vi "Elevator Bang Bang (before rewrite).vi"(8 "Hold Up Mode":bool, 9 "Top":bool, 10 "Middle":bool, 11 "Bottom":bool) -> (3 "in range":bool)   [LabVIEW 2014]
uses:
  Robot Global Data.vi
panel:
  out "Pot Value":dbl
  in  "Last Fed Value":dbl
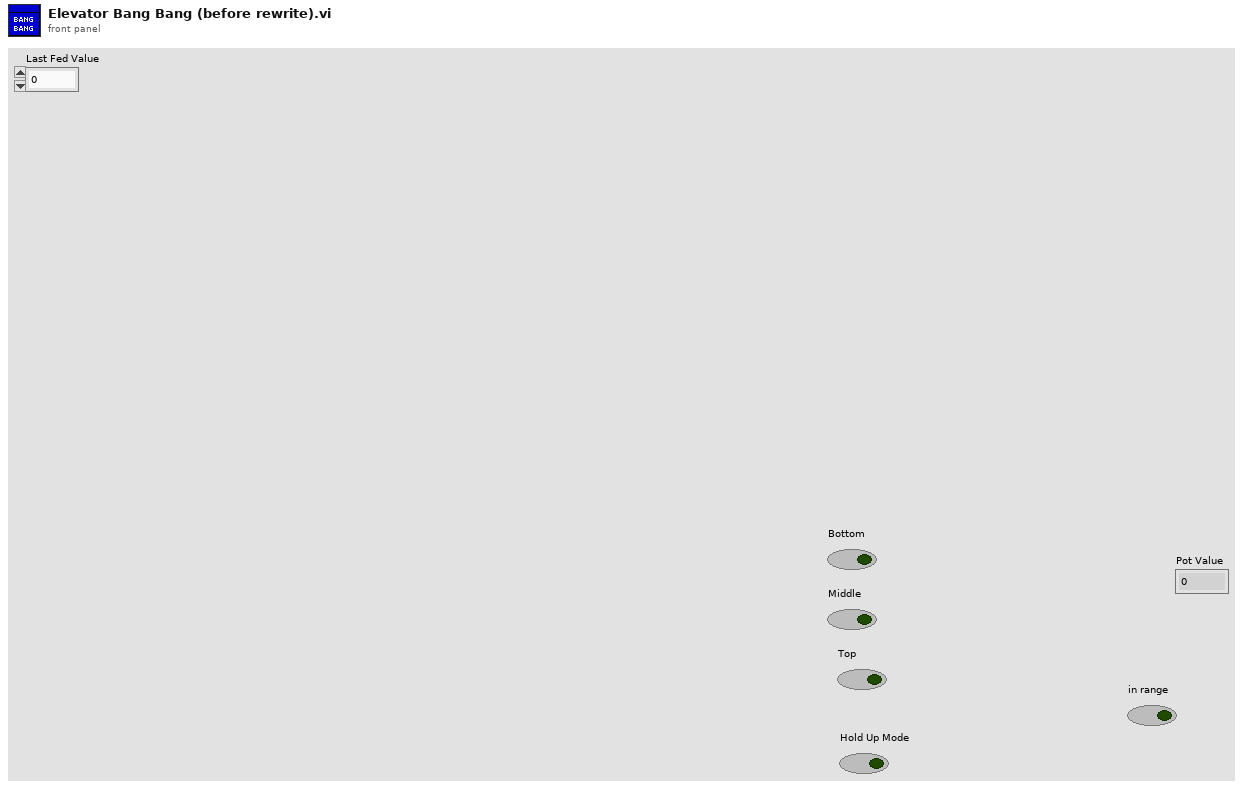
[diagram p1: front panel]
types:
  T1 = typedef "WPI_PotentiometerDevRef.ctl" = cluster{"DevStatus":errorcluster, "Controller":T2, "Analog Channel":T3, "Invert Output":bool}
  T2 = typedef "FPGA_TypedefAnalogModule.ctl" = enum16{"Controller 1"}
  T3 = typedef "FPGA_AIChannel.ctl" = enum8{"AI 0", "AI 1", "AI 2", "AI 3", "AI MXP 0", "AI MXP 1", "AI MXP 2", "AI MXP 3", "Invalid"}
  T4 = typedef "WPI_MotorControlDeviceRef.ctl" = cluster{"DeviceStatus":errorcluster, "Type":T5, "PWM":cluster{"Controller":T6, "PWM Channel":T7, "DeadBand":T8}, "CAN":cluster{"Device Number":u8, "Control Mode":T9, "Semaphore":T10, "Max Vout":dbl, "TalonSRX Control Mode":T11}, "Invert":bool, "TransformRef":T12, "InvTransformRef":T12}
  T5 = typedef "WPI_MotorControlType.ctl" = enum16{"PWM", "CAN", "CANTalonSRX"}
  T6 = typedef "FPGA_TypedefDigitalModule.ctl" = enum16{"Controller 1"}
  T7 = typedef "FPGA_DIOPWMChannel.ctl" = enum8{"PWM 0", "PWM 1", "PWM 2", "PWM 3", "PWM 4", "PWM 5", "PWM 6", "PWM 7", "PWM 8", "PWM 9", "PWM MXP 0", "PWM MXP 1", "PWM MXP 2", "PWM MXP 3", "PWM MXP 4", "PWM MXP 5", "PWM MXP 6", "PWM MXP 7", "PWM MXP 8", "PWM MXP 9", "Invalid"}
  T8 = typedef "WPI_PWMDeadband.ctl" = cluster{"Name":string, "maxPositivePwm":i32, "minPositivePwm":i32, "centerPwm":i32, "maxNegativePwm":i32, "minNegativePwm":i32, "angularRange":u16}
  T9 = typedef "WPI_CANJaguar_ControlMode.ctl" = enum8{"Percent VBus", "Current", "Speed", "Position", "Voltage"}
  T10 = typedef "Semaphore RefNum" = refnum<k1>
  T11 = typedef "WPI_CANTalonSRX_APIControlMode.ctl" = enum8{"Percent VBus", "Speed", "Position", "Slave", "Unchanged / Invalid"}
  T12 = typedef "WPI_PWMTransform_ConPane.ctl" = refnum<vi>
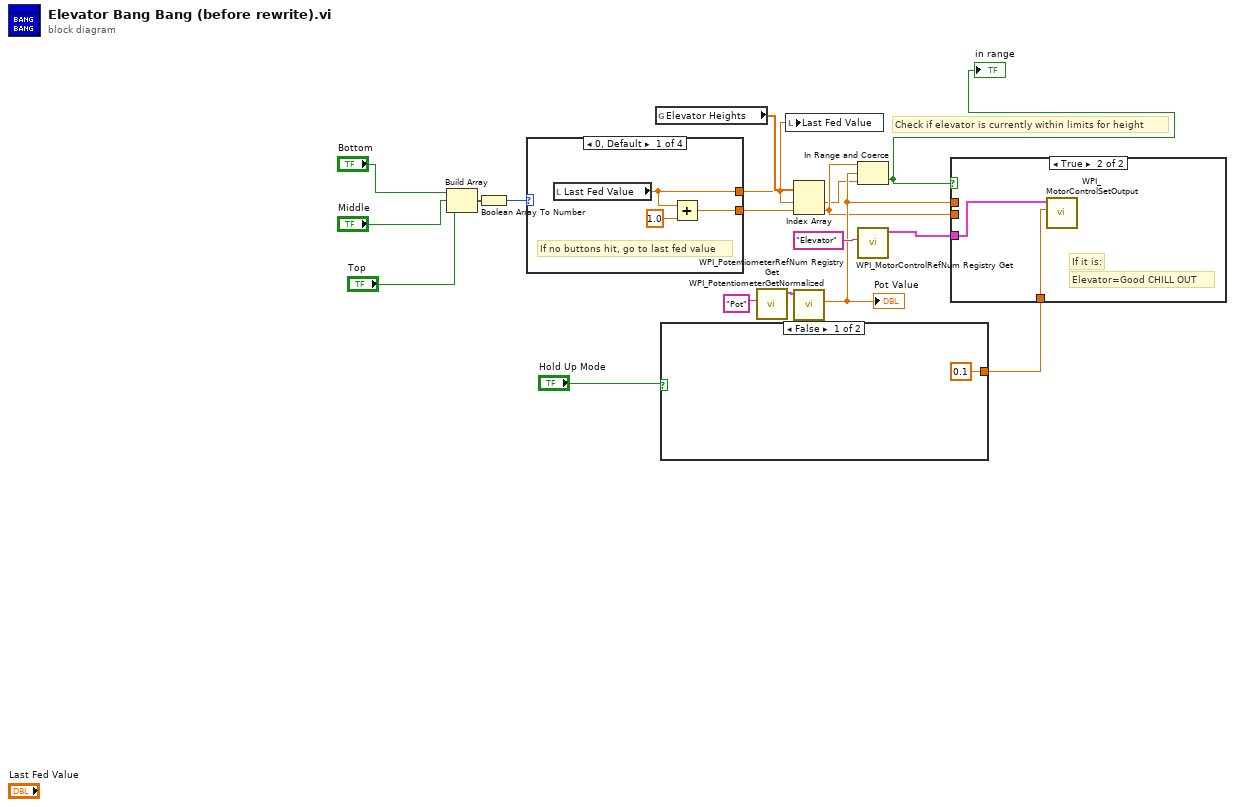
[diagram p0: block diagram]
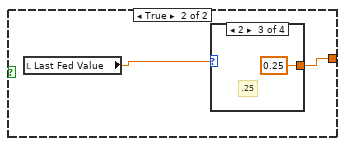
[diagram p2: hidden frame]
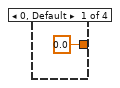
[diagram p3: hidden frame]
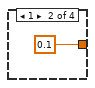
[diagram p4: hidden frame]
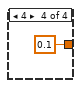
[diagram p5: hidden frame]
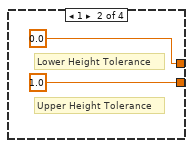
[diagram p6: hidden frame]
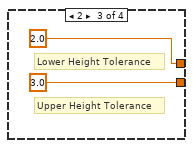
[diagram p7: hidden frame]
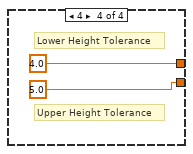
[diagram p8: hidden frame]
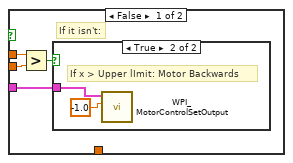
[diagram p9: hidden frame]
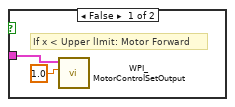
[diagram p10: hidden frame]
diagram:
  # "Check if elevator is currently within limits for height"
  n1 = Build Array("Bottom", "Middle", "Top") -> (w12:bool[])
  n2 = Boolean Array To Number(Boolean array=w12) -> (number=w2:u32)
  n3 = case shown="0, Default" w2 {
    tunnel: [w21 0.0 ("element") 2.0 ("element") 4.0 ("element")] -> w11
    tunnel: [w19 1.0 ("element") 3.0 ("element") 5.0 ("element")] -> w14
    frame 0, Default {
      # "If no buttons hit, go to last fed value"
      n4 = local read "Last Fed Value"() -> (w21:dbl)
      n5 = Add(x=w21, y=1.0) -> (x+y=w19:dbl)
    }
    frame 1 {
      # "Upper Height Tolerance"
      # "Lower Height Tolerance"
    }
    frame 2 {
      # "Upper Height Tolerance"
      # "Lower Height Tolerance"
    }
    frame 4 {
      # "Upper Height Tolerance"
      # "Lower Height Tolerance"
    }
  }
  n6 = global read "Robot Global Data.vi" "Elevator Heights"() -> (w15:dbl[])
  n7 = case shown="False" "Hold Up Mode" {
    tunnel: [0.1 ("Output") w30] -> w3
    frame False {
    }
    frame True {
      n8 = local read "Last Fed Value"() -> (w29:dbl)
      n9 = case shown="2" w29 {
        tunnel: [0.0 ("Output") 0.1 ("Output") 0.25 ("Output") 0.1 ("Output")] -> w30
        frame 0, Default {
        }
        frame 1 {
        }
        frame 2 {
          # ".25"
        }
        frame 4 {
        }
      }
    }
  }
  n10 = call <vilib>:"WPI_PotentiometerRefNum Registry Get.vi"("refnum name"="Pot") -> ("PotDevRef"=w18:T1)  [unwired: 9 in, 1 out]
  n11 = local write "Last Fed Value"(w11) -> ()
  n12 = Index Array(array=w15, index #1=w11, index #2=w14) -> (element #1=w4:dbl, element #2=w5:dbl)
  n13 = call <vilib>:"WPI_PotentiometerGetNormalized.vi"("PotDevRef"=w18) -> ("Normalized Value"=w10:dbl)  [unwired: 8 in, 2 out]
  "Pot Value" <- w10
  n14 = In Range and Coerce(upper limit=w5, x=w10, lower limit=w4) -> (In Range?=w6:bool)  [unwired: 1 out]
  "in range" <- w6
  n15 = call <vilib>:"WPI_MotorControlRefNum Registry Get.vi"("refnum name"="Elevator") -> ("MotorControlDevRef"=w13:T4)  [unwired: 9 in, 1 out]
  n16 = case shown="True" w6 {
    tunnel: w13 -> [w37 w44]
    tunnel: w10 -> [w36 _]
    tunnel: w5 -> [w35 _]
    tunnel: w3 -> [_ w43]
    frame False {
      # "If it isn't:"
      n17 = Greater?(x=w36, y=w35) -> (0:w38:bool)
      n18 = case shown="True" w38 {
        tunnel: w37 -> [w39 w41]
        frame False {
          # "If x < Upper lImit: Motor Forward"
          n19 = call <vilib>:"WPI_MotorControlSetOutput.vi"("Output"=1.0, "MotorControlDevRef"=w39) -> ()  [unwired: 7 in, 3 out]
        }
        frame True {
          # "If x > Upper lImit: Motor Backwards"
          n20 = call <vilib>:"WPI_MotorControlSetOutput.vi"("Output"=-1.0, "MotorControlDevRef"=w41) -> ()  [unwired: 7 in, 3 out]
        }
      }
    }
    frame True {
      # "If it is:"
      # "Elevator=Good CHILL OUT"
      n21 = call <vilib>:"WPI_MotorControlSetOutput.vi"("Output"=w43, "MotorControlDevRef"=w44) -> ()  [unwired: 7 in, 3 out]
    }
  }
